vi "R series Auger GUI.vi"() -> ()   [LabVIEW 2014]
uses:
  Count bar.ctl
  <vilib>/Utility/error.llb/Error Cluster From Error Code.vi
  <vilib>/rvi/errors/niLvFpgaAdjustHostInterfaceError.vi
  <vilib>/FPGAPlugInAG/PXI-7854R/niLvFpga_Close_PXI-7854R.vi
  <vilib>/rvi/interface/nirviReadWriteControl/nirviReadWriteControl.xnode
  FPGA Bitfiles/OmicronR2_FPGATarget_CountertoDAC_vJTICW5rMr0.lvbitx
  FPGA vi/Counter to DAC.vi
  <vilib>/rvi/interface/nirviMethod/nirviMethod.xnode
  <vilib>/rvi/interface/nirviCloseFPGA/nirviCloseFPGA.xnode
  <vilib>/rvi/errors/niLvFpgaMergeErrorWithErrorCode.vi
  NiFpgaLv.dll
  <vilib>/FPGAPlugInAG/PXI-7854R/niLvFpga_ReadFifo_PXI-7854R.vi
panel:
  in  "Hz per V1 [Hz]":dbl=500000.0 step=50000.0 format="%_3p"
  in  "Offset 1[Hz]":dbl min=-100000000.0 max=100000000.0 step=50000.0 format="%_3p"
  in  "Dac2 add":bool[](array[boolean])=[TRUE, TRUE, TRUE, TRUE, TRUE, TRUE, TRUE, FALSE]
  in  "Dac1 add":bool[](array[boolean])=[TRUE, TRUE, TRUE, TRUE, TRUE, TRUE, TRUE, FALSE]
  in  "Dac1 sub":bool[](array[boolean])=[FALSE, FALSE, FALSE, FALSE, FALSE, FALSE, FALSE, FALSE]
  in  "Dac2 sub":bool[](array[boolean])=[FALSE, FALSE, FALSE, FALSE, FALSE, FALSE, FALSE, FALSE]
  in  "DAC update [us]":u32=64 min=1 max=10000 step=1
  in  "Scale Delta":dbl=50000.0 min=1.0 max=100000000.0 step=1000.0 format="%#_3p"
  in  "Hz per V2 [Hz]":dbl=500000.0 step=50000.0 format="%_3p"
  in  "Offset 2[Hz]":dbl min=-100000000.0 max=100000000.0 step=50000.0 format="%_3p"
  out "DAC 1":sgl format="%.2f"
  out "DAC 2":sgl format="%.2f"
  in  "stop":bool
  in  "total scale":sgl=0.18 step=0.01
  out "index":i32
  in  "Time per point [s]":dbl=0.2 min=1e-06 max=4.0 step=0.01 format="%#_3p"
  out "Counts":T1={"C6"=0.0, "C4"=0.004405286, "C2"=0.008810572, "C1"=0.0, "C3"=0.0, "C5"=0.0, "C7"=0.0, "Max"=140000.0} {"Max" format="%#_2p"; "C7" scale=0.0..1.0; "C5" scale=0.0..1.0; "C3" scale=0.0..1.0; "C1" scale=0.0..1.0; "C2" scale=0.0..1.0; "C4" scale=0.0..1.0; "C6" scale=0.0..1.0}
  out "Graph":dbl[][](graph)
  in  "points":i32=300
  out "Count data":i32[][](array[numeric])
  in  "Timeout (ms)":i32=5000
  out "Counter ticks":u32
  out "FPGA error":errorcluster
  out "Ctr Actual":u32
  out "Ctr transfer":u32
  out "Last":i32[](array[numeric])
  out "Ctr Overflow?":bool
  out "loop count":i32
  # "set points to plot before start"
  # "Counts to Volts"
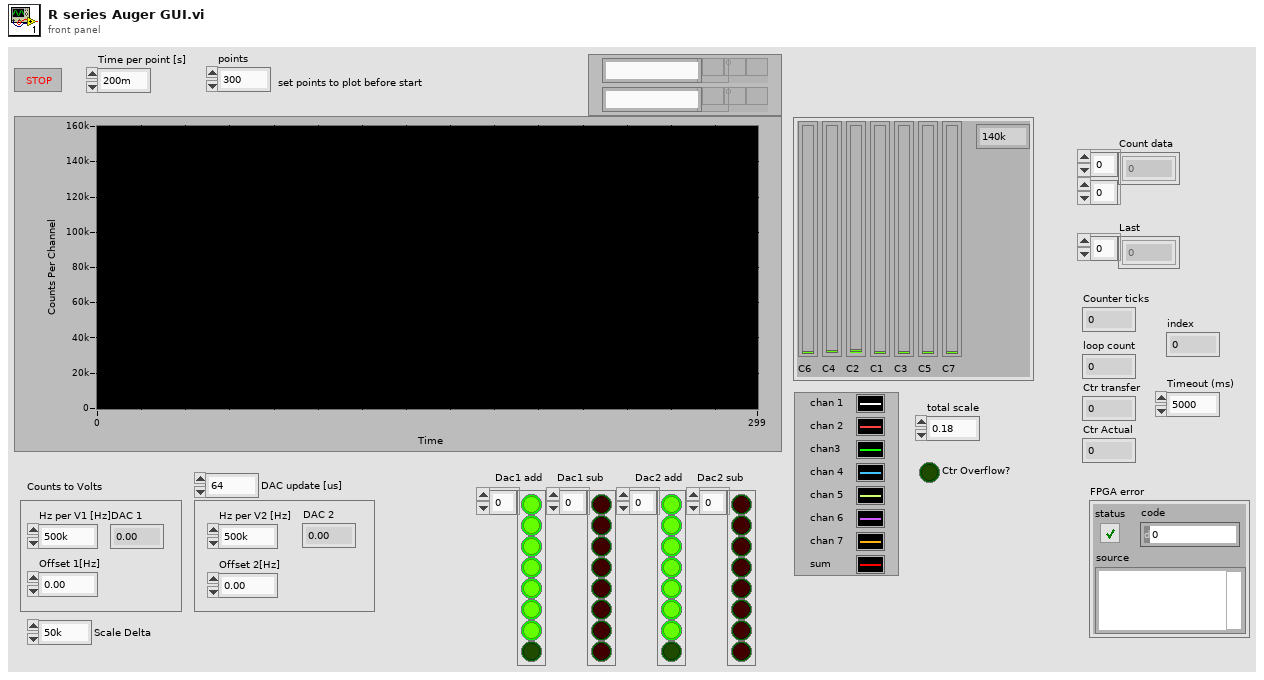
[diagram p1: front panel]
types:
  T1 = typedef "Count bar.ctl" = cluster{"C6":sgl, "C4":sgl, "C2":sgl, "C1":sgl, "C3":sgl, "C5":sgl, "C7":sgl, "Max":sgl}
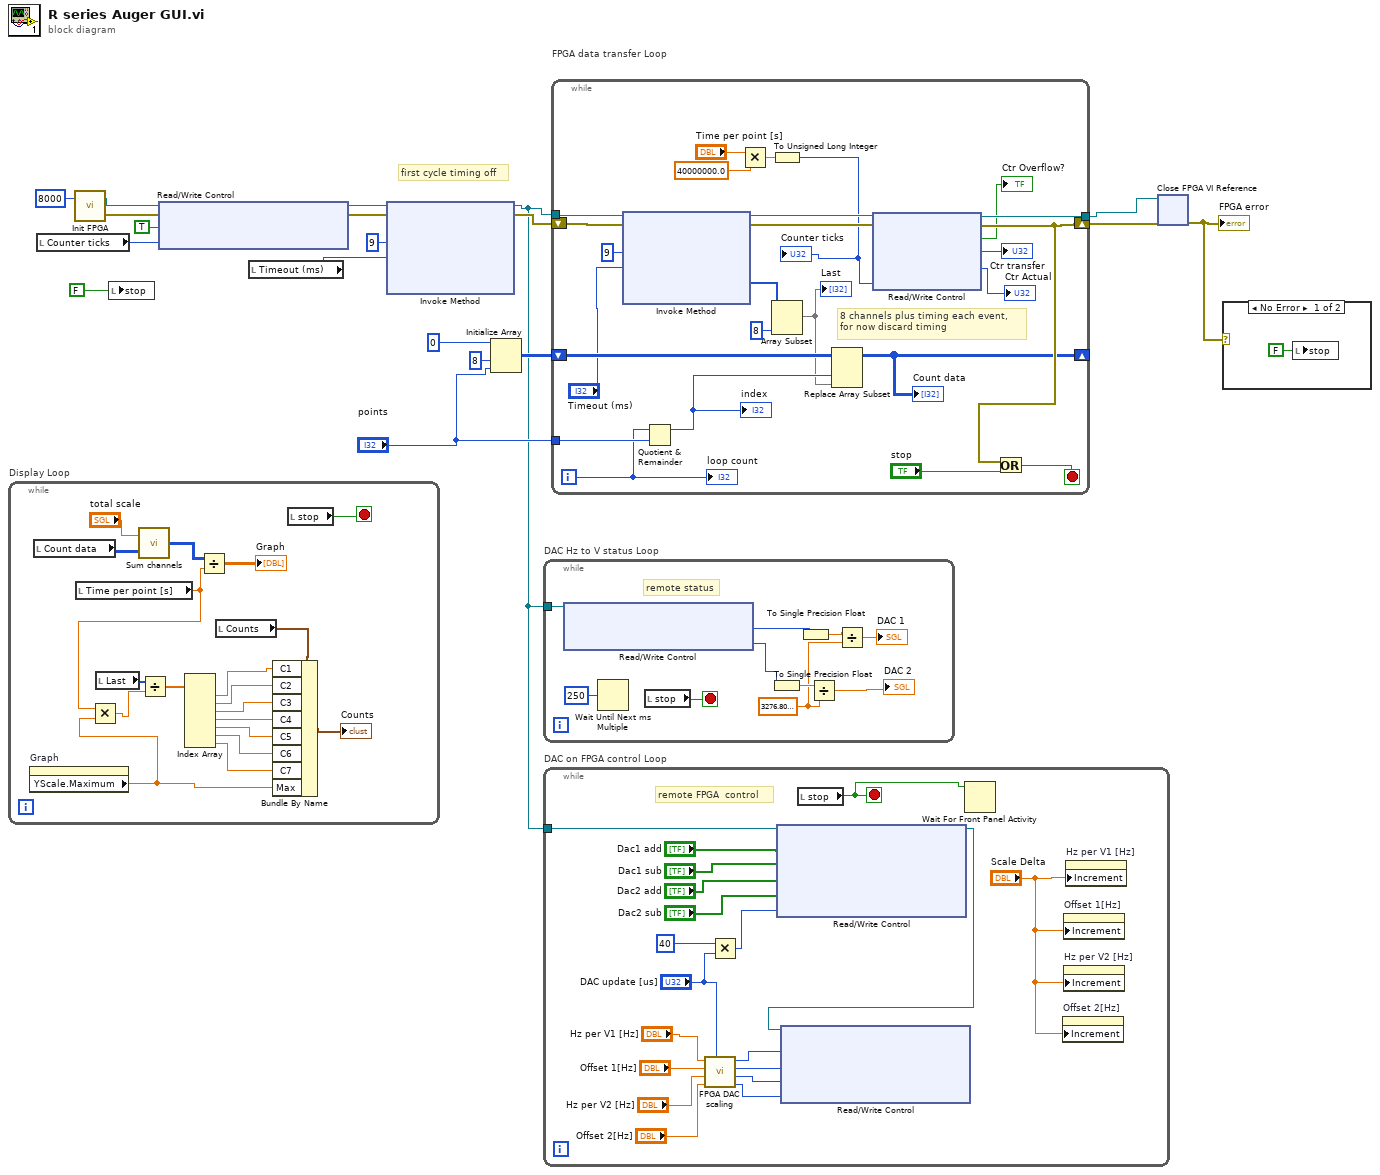
[diagram p0: block diagram]
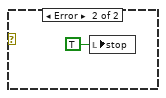
[diagram p2: hidden frame]
diagram:
  # "first cycle timing off"
  n1 = while "Display Loop" {
    stop <- w20 stop-if-true
    n2 = property on="Graph" class="WFGraph (strict)"() -> ("YScale.Maximum"=w25:dbl)  [unwired: 2 in, 2 out]
    n3 = local read "Count data"() -> (w23:i32[][])
    n4 = local read "Time per point [s]"() -> (w26:dbl)
    n5 = Multiply(x=w26, y=w25) -> (x*y=w27:dbl)
    n6 = local read "Last"() -> (w35:i32[])
    n7 = call "Sum channels.vi"("Count in"=w23, "scale"="total scale") -> ("Count out"=w22:i32[][])
    n8 = Divide(x=w35, y=w27) -> (x/y=w28:dbl[])
    n9 = Index Array(array=w28) -> (element #1=w36:dbl, element #2=w34:dbl, element #3=w33:dbl, element #4=w32:dbl, element #5=w31:dbl, element #6=w30:dbl, element #7=w29:dbl)  [unwired: 7 in]
    n10 = Divide(x=w22, y=w26) -> (x/y=→"Graph":dbl[][])
    n11 = local read "Counts"() -> (w38:T1)
    n12 = Bundle By Name(cluster=w38, "C1"=w36, "C2"=w34, "C3"=w33, "C4"=w32, "C5"=w31, "C6"=w30, "C7"=w29, "Max"=w25) -> (→"Counts":T1)
    n13 = local read "stop"() -> (w20:bool)
  }
  n14 = local read "Counter ticks"() -> (w9:u32)
  n15 = call "Init FPGA.vi"("FIFO depth"=u32 8000) -> ("FPGA error out"=w17:errorcluster, "FPGA VI Reference Out"=w18:refnum<k20>)  [unwired: 1 out]
  n16 = local write "stop"(FALSE ("stop")) -> ()
  n17 = xnode "Read/Write Control"("FPGA VI Reference In"=w18, "error in"=w17, "Ctr FIFO"=TRUE, "Counter ticks"=w9) -> ("FPGA VI Reference Out"=w7:refnum<k20>, "error out"=w6:errorcluster)
  n18 = local read "Timeout (ms)"() -> (w4:i32)
  n19 = xnode "Invoke Method"("FPGA VI Reference In"=w7, "error in"=w6, "Number of Elements"=u32 9, "Timeout (ms)"=w4) -> ("FPGA VI Reference Out"=w1:refnum<k20>, "error out"=w5:errorcluster)  [unwired: 2 out]
  n20 = Initialize Array(0 ("element"), 8 ("dimension size"), "points") -> (w13:i32[][])
  n21 = while "DAC Hz to V status Loop" {
    tunnel: w1 -> [w40]
    stop <- w39 stop-if-true
    w42 = sgl 3276.8 ("y")
    # "remote status"
    n22 = xnode "Read/Write Control"("FPGA VI Reference In"=w40) -> ("DAC 1"=w44:i16, "DAC 2"=w47:i16)  [unwired: 1 in, 2 out]
    n23 = Wait Until Next ms Multiple(millisecond multiple=u32 250) -> ()  [unwired: 1 out]
    n24 = local read "stop"() -> (w39:bool)
    n25 = To Single Precision Float(number=w47) -> (single precision float=w46:sgl)
    n26 = To Single Precision Float(number=w44) -> (single precision float=w43:sgl)
    n27 = Divide(x=w46, y=w42) -> (x/y=→"DAC 2":sgl)
    n28 = Divide(x=w43, y=w42) -> (x/y=→"DAC 1":sgl)
  }
  n29 = while "DAC on FPGA control Loop" {
    tunnel: w1 -> [w59]
    stop <- w49 stop-if-true
    # "remote FPGA  control"
    n30 = call "FPGA DAC scaling.vi"("DAC update [us]"="DAC update [us]", "Offset 2[Hz]"="Offset 2[Hz]", "Hz per V2 [Hz]"="Hz per V2 [Hz]", "Offset 1[Hz]"="Offset 1[Hz]", "Hz per V1 [Hz]"="Hz per V1 [Hz]") -> ("offset 2"=w54:i16, "scale 2"=w53:i16, "offset 1"=w52:i16, "scale 1"=w51:i16)  [unwired: 3 in]
    n31 = Multiply(x=u32 40 ("y"), y="DAC update [us]") -> (x*y=w62:u32)
    n32 = xnode "Read/Write Control"("FPGA VI Reference In"=w59, "Dac1 add"="Dac1 add", "Dac1 sub"="Dac1 sub", "Dac2 add"="Dac2 add", "Dac2 sub"="Dac2 sub", "Rate"=w62) -> ("FPGA VI Reference Out"=w60:refnum<k20>)  [unwired: 1 in, 1 out]
    n33 = xnode "Read/Write Control"("FPGA VI Reference In"=w60, "Scale 1"=w51, "Offset 1"=w52, "Scale 2"=w53, "Offset 2"=w54) -> ()  [unwired: 1 in, 2 out]
    n34 = local read "stop"() -> (w49:bool)
    n35 = Wait For Front Panel Activity(3:w49) -> ()  [unwired: 2 in, 1 out]
    n36 = property on="Offset 2[Hz]" class="DigNum (strict)"("Increment"="Scale Delta") -> ()  [unwired: 2 in, 2 out]
    n37 = property on="Offset 1[Hz]" class="DigNum (strict)"("Increment"="Scale Delta") -> ()  [unwired: 2 in, 2 out]
    n38 = property on="Hz per V2 [Hz]" class="DigNum (strict)"("Increment"="Scale Delta") -> ()  [unwired: 2 in, 2 out]
    n39 = property on="Hz per V1 [Hz]" class="DigNum (strict)"("Increment"="Scale Delta") -> ()  [unwired: 2 in, 2 out]
  }
  n40 = while "FPGA data transfer Loop" {
    tunnel: w1 -> [w92]
    shift-right: [w82] -> w12
    shift-left: w5 -> [w91]
    tunnel: [w87] -> w11
    shift-right: [w81] -> _
    shift-left: w13 -> [w90]
    tunnel: "points" -> [w80]
    i -> [w79]
    stop <- w84 stop-if-true
    # "8 channels plus timing each event, \nfor now discard timing"
    n41 = xnode "Invoke Method"("FPGA VI Reference In"=w92, "error in"=w91, "Number of Elements"=u32 9, "Timeout (ms)"="Timeout (ms)") -> ("FPGA VI Reference Out"=w89:refnum<k20>, "error out"=w88:errorcluster, "Data"=w70:u32[])  [unwired: 1 out]
    n42 = Quotient & Remainder(x=w79, y=w80) -> (x-y*floor(x/y)=w78:i32)  [unwired: 1 out]
    "index" <- w78
    n43 = Multiply(x="Time per point [s]", y=40000000.0) -> (x*y=w75:dbl)
    n44 = To Unsigned Long Integer(number=w75) -> (unsigned 32bit integer=w74:u32)
    "Counter ticks" <- w74
    n45 = Array Subset(array=w70, length=8) -> (w68:u32[])  [unwired: 1 in]
    "Last" <- w68
    n46 = Replace Array Subset(array=w90, new element=w68, index (col)=w78) -> (w81:i32[][])  [unwired: 1 in]
    "Count data" <- w81
    n47 = xnode "Read/Write Control"("FPGA VI Reference In"=w89, "error in"=w88, "Counter ticks"=w74) -> ("FPGA VI Reference Out"=w87:refnum<k20>, "error out"=w82:errorcluster, "Ctr Overflow?"=→"Ctr Overflow?":bool, "BlocksTransfered"=→"Ctr transfer":u32, "Ctr Elapsed"=→"Ctr Actual":u32)
    n48 = Or(x=w82, y="stop") -> (x .or. y?=w84:bool)
    "loop count" <- w79
  }
  n49 = xnode "Close FPGA VI Reference"("FPGA VI Reference In"=w11, "error in"=w12) -> ("error out"=w2:errorcluster)
  "FPGA error" <- w2
  n50 = case shown="No Error" w2 {
    frame No Error {
      n51 = local write "stop"(FALSE ("stop")) -> ()
    }
    frame Error {
      (unwired) FALSE ("stop")
      (unwired) FALSE ("stop")
      (unwired) FALSE ("stop")
      n52 = local write "stop"(TRUE ("stop")) -> ()
    }
  }
